vi "Determine Warning.vi"() -> ()   [LabVIEW 2014]
panel:
  out "error out":errorcluster
  in  "error in (no error)":errorcluster
  in  "Min Temp 2":dbl
  out "Warning":bool
  out "Warning Tex":string
  in  "Max temp":dbl
  in  "Current Temp":dbl
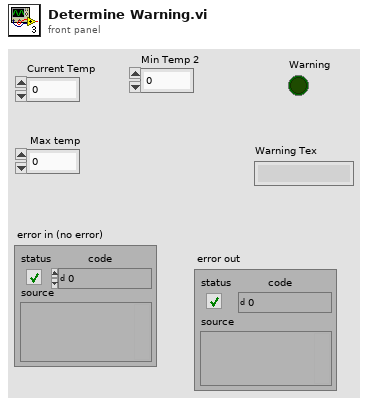
[diagram p1: front panel]
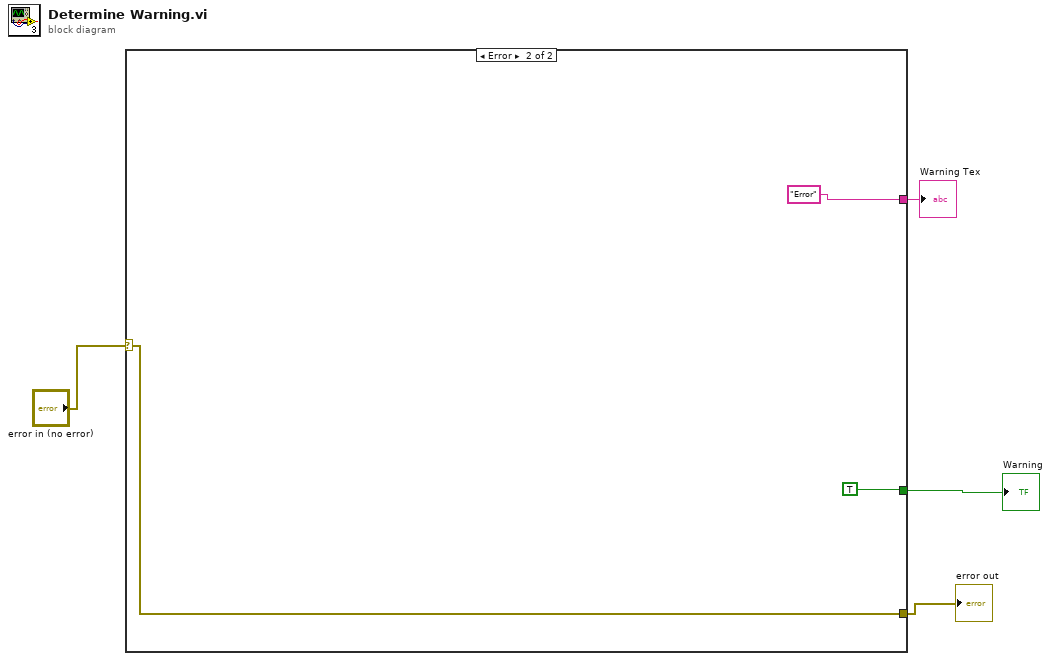
[diagram p0: block diagram]
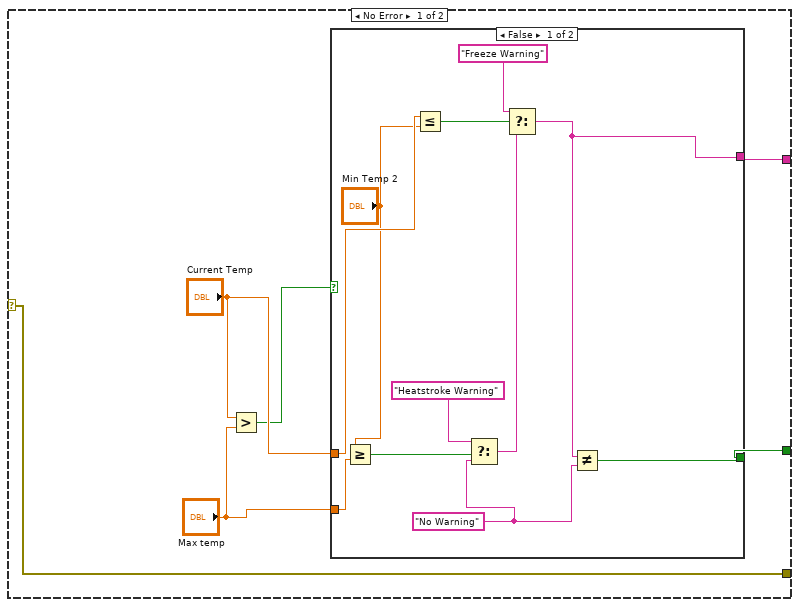
[diagram p2: hidden frame]
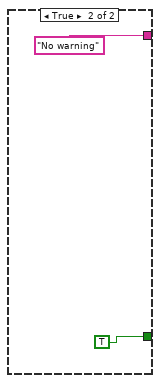
[diagram p3: hidden frame]
diagram:
  n1 = case shown="Error" "error in (no error)" {
    selector: "error in (no error)" -> [w5 w26]
    tunnel: [w10 TRUE ("Warning")] -> w4
    tunnel: [w9 "Error" ("Warning Tex")] -> w3
    tunnel: [w5 w26] -> w1
    frame No Error {
      n2 = Greater?(x="Current Temp", y="Max temp") -> (0:w6:bool)
      n3 = case shown="False" w6 {
        tunnel: "Current Temp" -> [w12 _]
        tunnel: "Max temp" -> [w13 _]
        tunnel: [w14 TRUE] -> w10
        tunnel: [w15 "No warning"] -> w9
        frame False {
          w19 = "No Warning"
          n4 = Greater Or Equal?(x="Min Temp 2", y=w13) -> (x >= y?=w20:bool)
          n5 = Less Or Equal?(x=w12, y="Min Temp 2") -> (x <= y?=w17:bool)
          n6 = Select(t="Heatstroke Warning", s=w20, f=w19) -> (s? t:f=w18:string)
          n7 = Select(t="Freeze Warning", s=w17, f=w18) -> (s? t:f=w15:string)
          n8 = Not Equal?(x=w15, y=w19) -> (x != y?=w14:bool)
        }
        frame True {
        }
      }
    }
    frame Error {
    }
  }
  "Warning Tex" <- w3
  "Warning" <- w4
  "error out" <- w1
